vi "Start Saw.vi"(8 "error in (no error)":errorcluster, 11 "Logging in":refnum<class "Logging.lvclass">) -> (0 "error out":errorcluster, 3 "State Machine Actor out":refnum<class "State Machine Actor.lvclass">)   [LabVIEW 2024, in "Logging.lvlib" / "Logging.lvclass"]
uses:
  Logging.lvclass
  C:/Users/uspoaotto/OneDrive - Oregon Tool/Desktop/working copies/stateMachineActor/src/State Machine Actor/State Machine Actor/State Machine Actor.lvclass
  State Machine Actor/State Machine Actor/State Machine Actor.lvclass
  Saw Running/Saw Running/Saw Running.lvclass
  Logging.lvclass/Logging.ctl
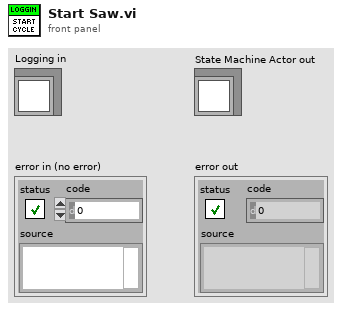
[diagram p1: front panel]
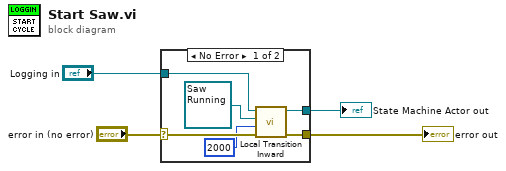
[diagram p0: block diagram]
diagram:
  n1 = case shown="No Error" "error in (no error)" {
    selector: "error in (no error)" -> [w8 w11]
    tunnel: "Logging in" -> [w10 w12]
    tunnel: [w7 w11] -> w2
    tunnel: [w6 w12] -> w1
    frame No Error {
      n2 = call-dynamic "Local Transition Inward.vi"("error in (no error)"=w8, "Timeout Period in ms (-1, never)"=2000, "Target State in"=refnum<class "Saw Running.lvclass"> refnum ("Saw Running.lvlib:Saw Running.lvclass"), "State Machine Actor in"=w10) -> ("error out"=w7:errorcluster, "State Machine Actor out"=w6:refnum<class "State Machine Actor.lvclass">)  [unwired: 6 in]
    }
    frame Error {
    }
  }
  "error out" <- w2
  "State Machine Actor out" <- w1
